vi "CalcPiezoValues.vi"(2 "Tilt":dbl, 3 "A2":dbl, 4 "A1":dbl, 5 "Rotator Position":dbl) -> (0 "Right Piezo":i32, 1 "Left Piezo":i32)   [LabVIEW 2015]
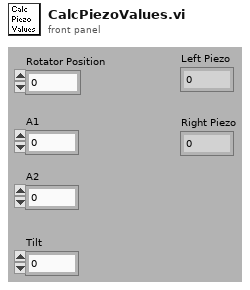
[diagram p1: front panel]
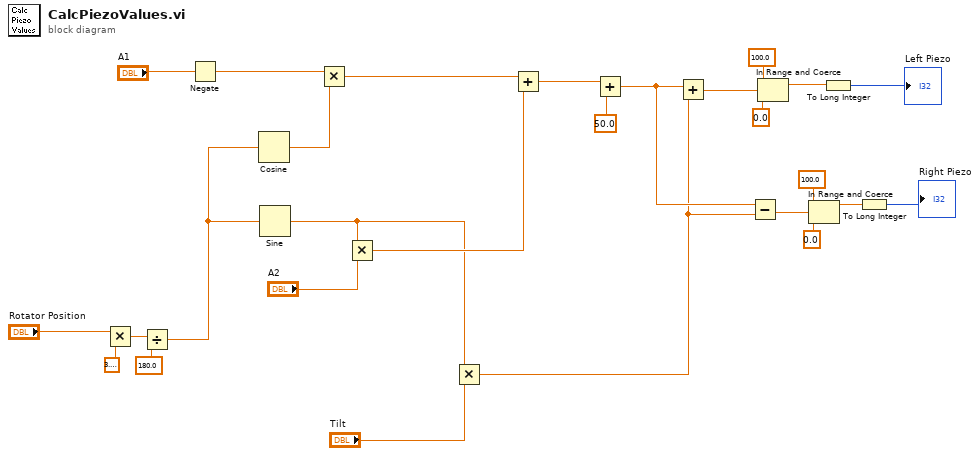
[diagram p0: block diagram]
diagram:
  n1 = Multiply(x="Rotator Position", y=3.141592653589793) -> (x*y=w24:dbl)
  n2 = Divide(x=w24, y=180.0) -> (x/y=w19:dbl)
  n3 = Negate(x="A1") -> (-x=w22:dbl)
  n4 = Cosine(x=w19) -> (cos(x)=w21:dbl)
  n5 = Sine(x=w19) -> (sin(x)=w14:dbl)
  n6 = Multiply(x=w22, y=w21) -> (x*y=w20:dbl)
  n7 = Multiply(x=w14, y="A2") -> (x*y=w17:dbl)
  n8 = Multiply(x=w14, y="Tilt") -> (x*y=w11:dbl)
  n9 = Add(x=w20, y=w17) -> (x+y=w16:dbl)
  n10 = Add(x=w16, y=50.0) -> (x+y=w12:dbl)
  n11 = Add(x=w12, y=w11) -> (x+y=w10:dbl)
  n12 = Subtract(x=w12, y=w11) -> (x-y=w5:dbl)
  n13 = In Range and Coerce(upper limit=100.0, x=w10, lower limit=0.0) -> (coerced(x)=w4:dbl)  [unwired: 1 out]
  n14 = In Range and Coerce(upper limit=100.0, x=w5, lower limit=0.0) -> (coerced(x)=w3:dbl)  [unwired: 1 out]
  n15 = To Long Integer(number=w4) -> (32bit integer=→"Left Piezo":i32)
  n16 = To Long Integer(number=w3) -> (32bit integer=→"Right Piezo":i32)
